vi "Disconnect.vi"(8 "error in":errorcluster, 11 "ManualPS in":refnum<class "ManualPS.lvclass">) -> (0 "error out":errorcluster, 3 "ManualPS out":refnum<class "ManualPS.lvclass">)   [LabVIEW 2018, in "ManualPS.lvlib" / "ManualPS.lvclass"]
uses:
  ManualPS.lvclass
panel:
  in  "OK Button":bool
  # "Verify power supply is turned off"
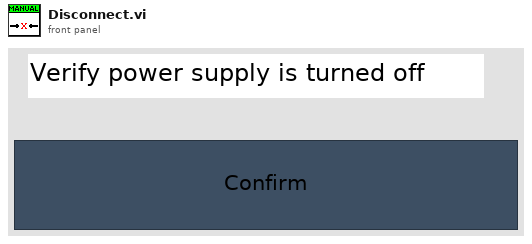
[diagram p1: front panel]
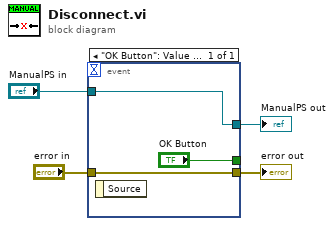
[diagram p0: block diagram]
diagram:
  n1 = event shown="[0] \"OK Button\": Value Change" {
    selector: _ -> [_]
    dyn-events: _ -> [_]
    timeout: _ -> [_]
    tunnel: "ManualPS in" -> [w6]
    tunnel: "error in" -> [w7]
    tunnel: [w7] -> w1
    tunnel: [w6] -> w2
    tunnel: ["OK Button"] -> _
    event "OK Button": Value Change {
      n2 = event-data() -> ()  [unwired: 1 in, 1 out]
    }
  }
  "error out" <- w1
  "ManualPS out" <- w2
